vi "Recursive Search and Replace.vi"(8 "error in (no error)":errorcluster, 9 "Replacement Log In":string[](array[string]), 10 "Replacement Channels":T1={"Channel to Replace"="Targets/Controller/Custom Devices/VCOM/CAN_Sender_Tx/ACC/ACC_ESP_E2E_PR2/ACC_NEW_SIGNAL", "Replacement Channel"="Targets/Controller/User Channels/User Channel 1"}, 11 "Reference In":refnum<k24>) -> (0 "error out":errorcluster, 3 "Replacement Log":string[](array[string]))   [LabVIEW 2025]
uses:
  NationalInstruments.VeriStand.SystemDefinitionAPI
  Controls/Replacement Channels.ctl
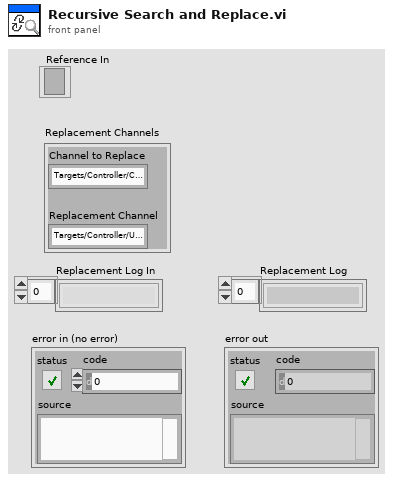
[diagram p1: front panel]
types:
  T1 = typedef "Replacement Channels.ctl" = cluster{"Channel to Replace":string, "Replacement Channel":string}
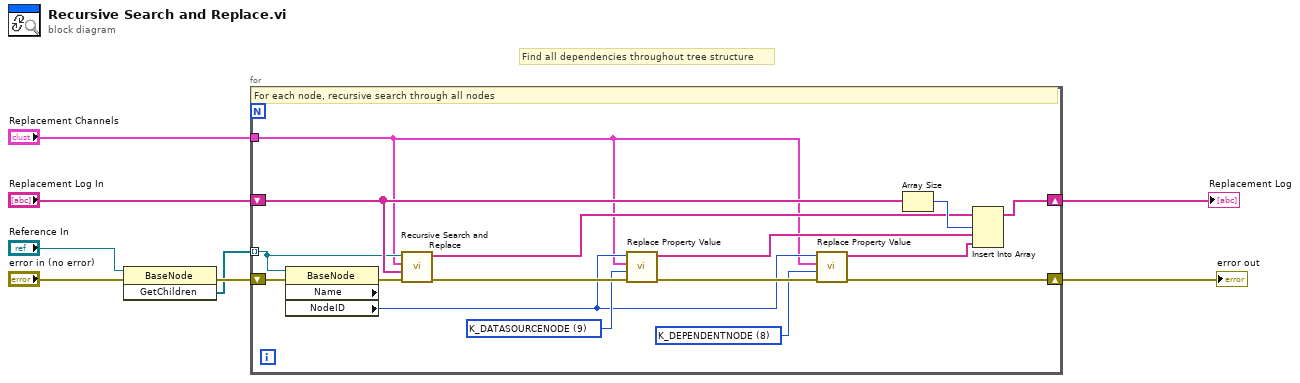
[diagram p0: block diagram]
diagram:
  # "Find all dependencies throughout tree structure"
  n1 = invoke class="BaseNode" method="GetChildren"(reference="Reference In", error in="error in (no error)") -> (error out=w7:errorcluster, "GetChildren"=w1:refnum<k24>[])  [unwired: 1 in, 1 out]
  n2 = for {
    shift-right: [w14] -> w5
    shift-left: w7 -> [w24]
    shift-right: [w22] -> w4
    shift-left: "Replacement Log In" -> [w21]
    tunnel: "Replacement Channels" -> [w9]
    tunnel: w1 -> [w12] mode=indexing
    w16 = 8 items=["K_STRING", "K_BOOL", "K_I32", "K_U32", "K_DOUBLE", "K_U64", "K_VARIANT", "K_DEPENDENTFILE", "K_DEPENDENTNODE", "K_DATASOURCENODE", "K_U16", "K_DBLARR", "K_U32ARR", "K_I32ARR", "K_STRINGARR", "K_DICTIONARY", "K_DICTIONARYARR", "K_BINARYSTRING", "K_I16", "K_I64", "K_BOOLARR", "K_U64ARR", "K_U16ARR", "K_I64ARR", "K_I16ARR"] ("Property Type")
    w18 = 9 items=["K_STRING", "K_BOOL", "K_I32", "K_U32", "K_DOUBLE", "K_U64", "K_VARIANT", "K_DEPENDENTFILE", "K_DEPENDENTNODE", "K_DATASOURCENODE", "K_U16", "K_DBLARR", "K_U32ARR", "K_I32ARR", "K_STRINGARR", "K_DICTIONARY", "K_DICTIONARYARR", "K_BINARYSTRING", "K_I16", "K_I64", "K_BOOLARR", "K_U64ARR", "K_U16ARR", "K_I64ARR", "K_I16ARR"] ("Property Type")
    # "For each node, recursive search through all nodes"
    n3 = property class="BaseNode" props=["Name", "NodeID"](reference=w12, error in=w24) -> (error out=w11:errorcluster, "NodeID"=w15:u64)  [unwired: 2 out]
    n4 = call "Recursive Search and Replace.vi"("error in (no error)"=w11, "Replacement Log In"=w21, "Replacement Channels"=w9, "Reference In"=w12) -> ("error out"=w19:errorcluster, "Replacement Log"=w10:string[])  [unwired: 6 in]
    n5 = call "Replace Property Value.vi"("error in (no error)"=w19, "Property Type"=w18, "Replacement Channels"=w9, "NodeID"=w15) -> ("error out"=w17:errorcluster, "Replacement Log"=w20:string[])  [unwired: 6 in]
    n6 = call "Replace Property Value.vi"("error in (no error)"=w17, "Property Type"=w16, "Replacement Channels"=w9, "NodeID"=w15) -> ("error out"=w14:errorcluster, "Replacement Log"=w13:string[])  [unwired: 6 in]
    n7 = Array Size(array=w21) -> (size(s)=w23:i32)
    n8 = Insert Into Array(array=w10, index=w23, new element #1=w20, new element #2=w13) -> (w22:string[])
  }
  "error out" <- w5
  "Replacement Log" <- w4
